vi "Cargo State Control.vi"(9 "Elevator State":string) -> ()   [LabVIEW 2018]
uses:
  RefNumsDriverStation.vi
  Robot States.vi
  Motor Power.vi
  Sensor Readings.vi
panel:
  out "CargoCapturedTest":bool
  in  "Current currewnt value":dbl=30.0
  out "Intake Velocity":dbl
  in  "Threshold (ms)":u32=300
  in  "Current Threshold (A)":dbl=20.0
  in  "Current Ignore Time  (ms)":u32=1000
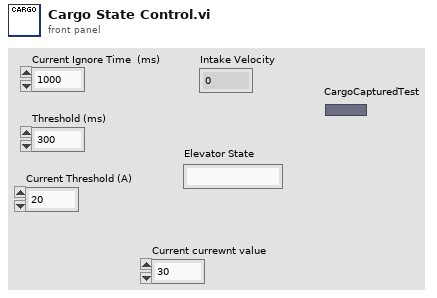
[diagram p1: front panel]
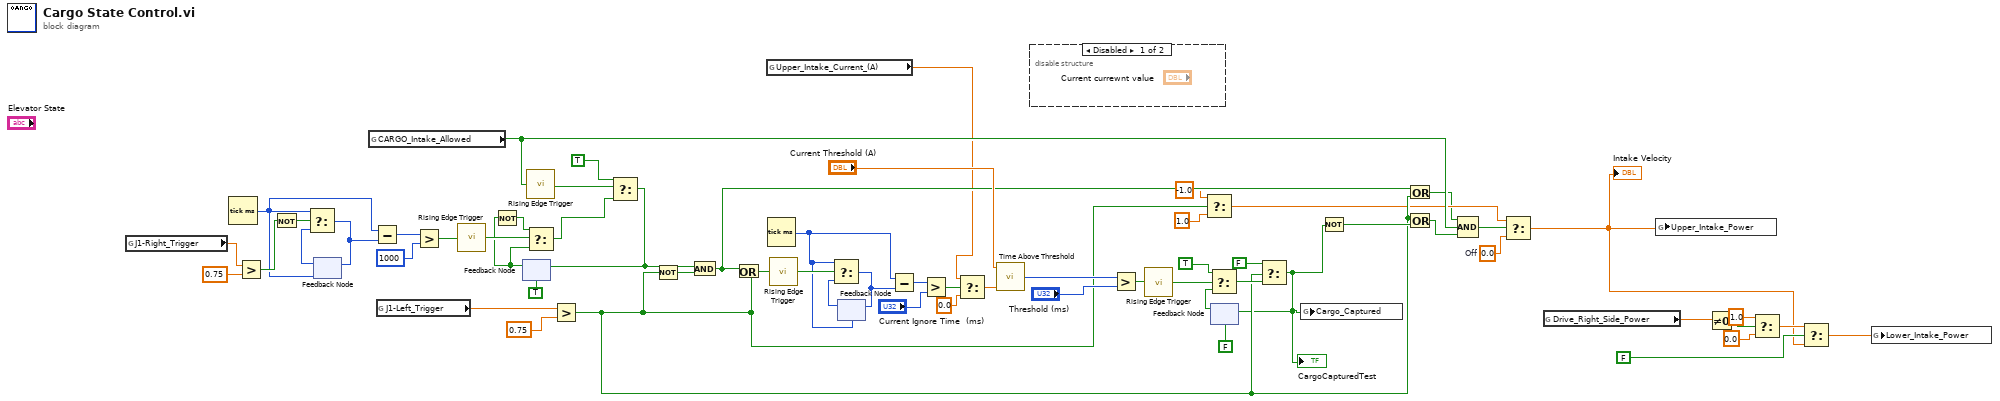
[diagram p0: block diagram]
diagram:
  w15 = 0.0  # Off
  n1 = global read "RefNumsDriverStation.vi" "J1-Right_Trigger"() -> (w46:dbl)
  n2 = Tick Count (ms)() -> (millisecond timer value=w57:u32)
  n3 = Greater?(x=w46, y=0.75) -> (0:w61:bool)
  n4 = Not(x=w61) -> (.not. x?=w62:bool)
  n5 = feedback #1(w57) -> (w59:u32)
  n6 = Select(t=w57, s=w62, f=w59) -> (s? t:f=w58:u32)
  n7 = feedback-in #1(w58) -> ()
  n8 = global read "Robot States.vi" "CARGO_Intake_Allowed"() -> (w21:bool)
  n9 = Subtract(x=w57, y=w58) -> (x-y=w56:u32)
  n10 = global read "RefNumsDriverStation.vi" "J1-Left_Trigger"() -> (w45:dbl)
  n11 = Greater?(x=w56, y=u32 1000) -> (0:w54:bool)
  n12 = call "Rising Edge Trigger.vi"("Raw Signal"=w54) -> ("Trigger"=w53:bool)
  n13 = feedback #2(TRUE ("t")) -> (w47:bool)
  n14 = Not(x=w47) -> (.not. x?=w52:bool)
  n15 = call "Rising Edge Trigger.vi"("Raw Signal"=w21) -> ("Trigger"=w49:bool)
  n16 = Select(t=w52, s=w53, f=w47) -> (s? t:f=w51:bool)
  n17 = Greater?(x=w45, y=0.75) -> (0:w19:bool)
  n18 = Select(t=TRUE, s=w49, f=w51) -> (s? t:f=w42:bool)
  n19 = feedback-in #2(w42) -> ()
  n20 = Not(x=w19) -> (.not. x?=w43:bool)
  n21 = And(x=w42, y=w43) -> (x .and. y?=w22:bool)
  n22 = Or(x=w22, y=w19) -> (x .or. y?=w41:bool)
  n23 = global read "Sensor Readings.vi" "Upper_Intake_Current_(A)"() -> (w1:dbl)
  n24 = Tick Count (ms)() -> (millisecond timer value=w6:u32)
  n25 = call "Rising Edge Trigger.vi"("Raw Signal"=w41) -> ("Trigger"=w40:bool)
  n26 = feedback #3(w6) -> (w5:u32)
  n27 = Select(t=w6, s=w40, f=w5) -> (s? t:f=w39:u32)
  n28 = feedback-in #3(w39) -> ()
  n29 = Subtract(x=w6, y=w39) -> (x-y=w38:u32)
  n30 = Greater?(x=w38, y="Current Ignore Time  (ms)") -> (0:w37:bool)
  n31 = Select(t=w1, s=w37, f=0.0) -> (s? t:f=w34:dbl)
  n32 = call "Time Above Threshold.vi"("Current Value"=w34, "Threshold"="Current Threshold (A)") -> ("Time Above"=w32:u32)  [unwired: 3 in]
  n33 = disable-structure shown="Disabled" {
    frame Disabled {
    }
    frame Enabled {
    }
  }
  n34 = Greater?(x=w32, y="Threshold (ms)") -> (0:w30:bool)
  n35 = call "Rising Edge Trigger.vi"("Raw Signal"=w30) -> ("Trigger"=w29:bool)
  n36 = Select(t=-1.0, s=w19, f=1.0) -> (s? t:f=w16:dbl)
  n37 = feedback #4(FALSE) -> (w25:bool)
  n38 = Select(t=TRUE, s=w29, f=w25) -> (s? t:f=w27:bool)
  n39 = Select(t=FALSE, s=w19, f=w27) -> (s? t:f=w2:bool)
  "CargoCapturedTest" <- w2
  n40 = feedback-in #4(w2) -> ()
  n41 = global write "Sensor Readings.vi" "Cargo_Captured"(w2) -> ()
  n42 = Not(x=w2) -> (.not. x?=w23:bool)
  n43 = Or(x=w22, y=w19) -> (x .or. y?=w4:bool)
  n44 = Or(x=w19, y=w23) -> (x .or. y?=w3:bool)
  n45 = Compound Arithmetic op=AND(w4, w21, w3) -> (w20:bool)
  n46 = Select(t=w16, s=w20, f=w15) -> (s? t:f=w8:dbl)
  "Intake Velocity" <- w8
  n47 = global read "Motor Power.vi" "Drive_Right_Side_Power"() -> (w14:dbl)
  n48 = global write "Motor Power.vi" "Upper_Intake_Power"(w8) -> ()
  n49 = Not Equal To 0?(x=w14) -> (x != 0?=w13:bool)
  n50 = Select(t=1.0, s=w13, f=0.0) -> (s? t:f=w10:dbl)
  n51 = Select(t=w10, s=FALSE, f=w8) -> (s? t:f=w7:dbl)
  n52 = global write "Motor Power.vi" "Lower_Intake_Power"(w7) -> ()
